vi "He3_Tlogger_Global 1.vi"() -> ()   [LabVIEW 2013]
panel:
  in  "elapsed time (s)":dbl
  in  "Sorb (sensor A) (K)":dbl
  in  "Sample (sensor B) (K)":dbl
  in  "1K pot (sensor A) (K)":dbl
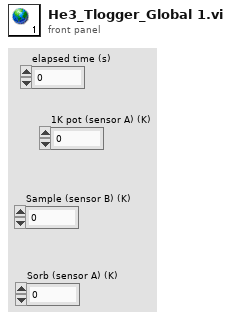
[diagram p1: front panel]
diagram:
